vi "EV05故障解析.vi"() -> ()   [LabVIEW 2013]
panel:
  in  "选择故障类型":u32(ring) items=["电池故障", "硬件故障", "电池系统故障1", "电池系统故障2"]
  in  "输入故障码":string
  in  "故码障解析123":bool
  out "电池故障":string[][](array[string])
  # "故障码解析"
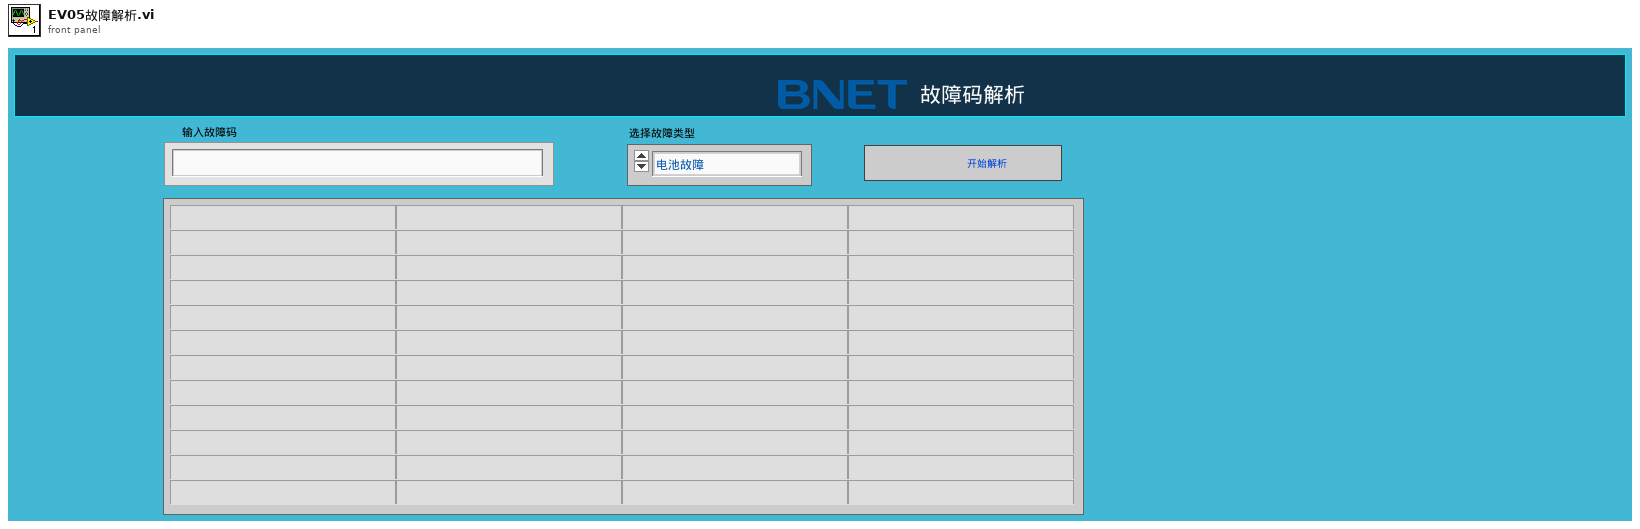
[diagram p1: front panel]
types:
  T1 = enum32{"Invalid", "Standard", "Closed", "Hidden", "Minimized", "Maximized"}
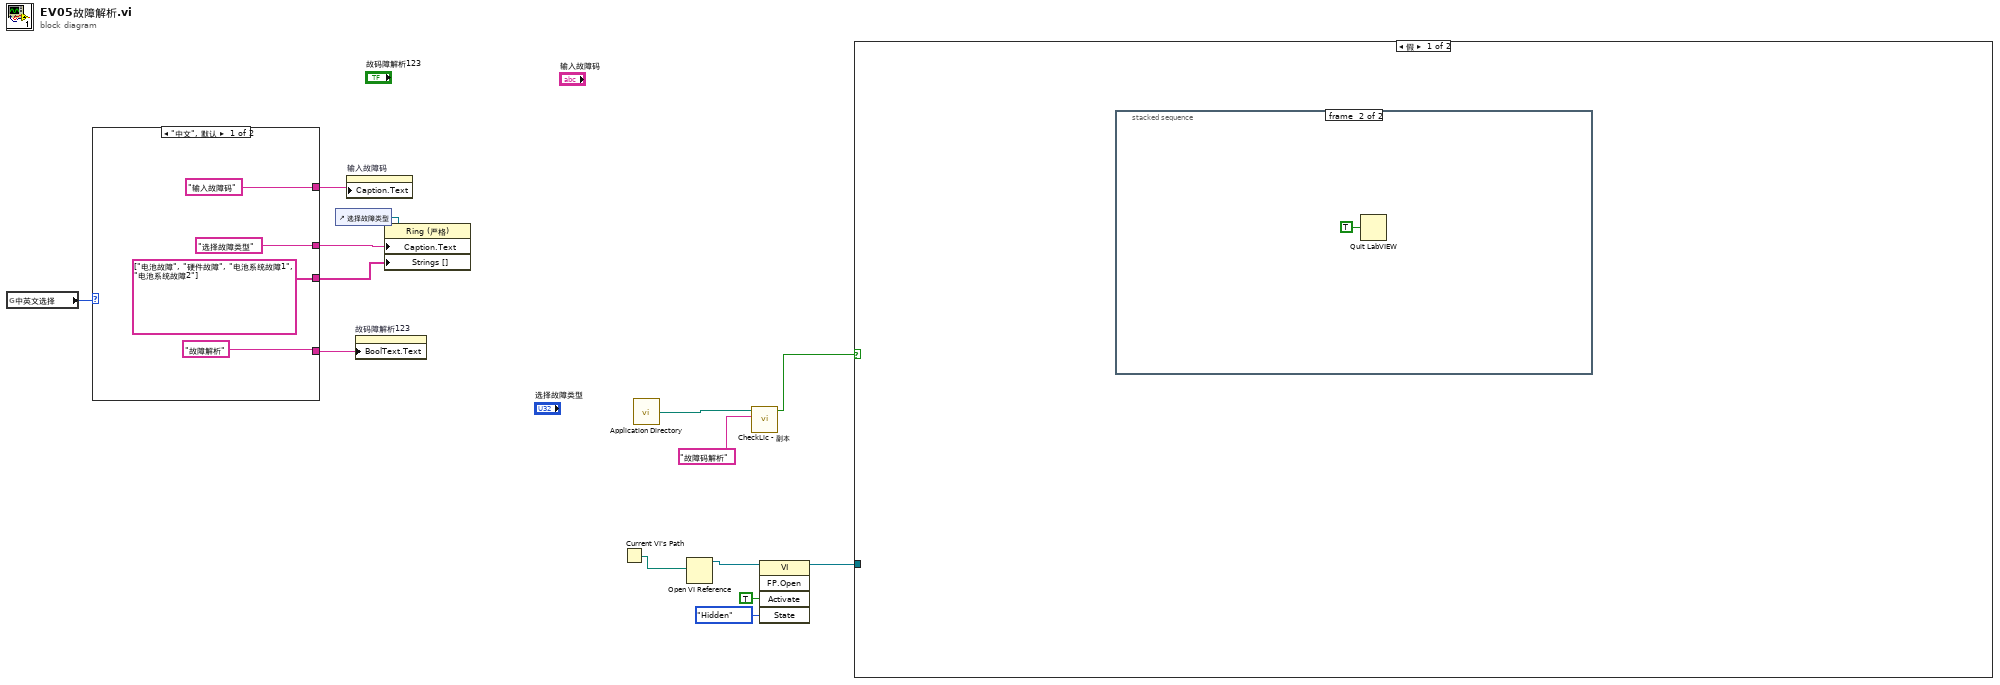
[diagram p0: block diagram]
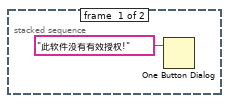
[diagram p2: hidden frame]
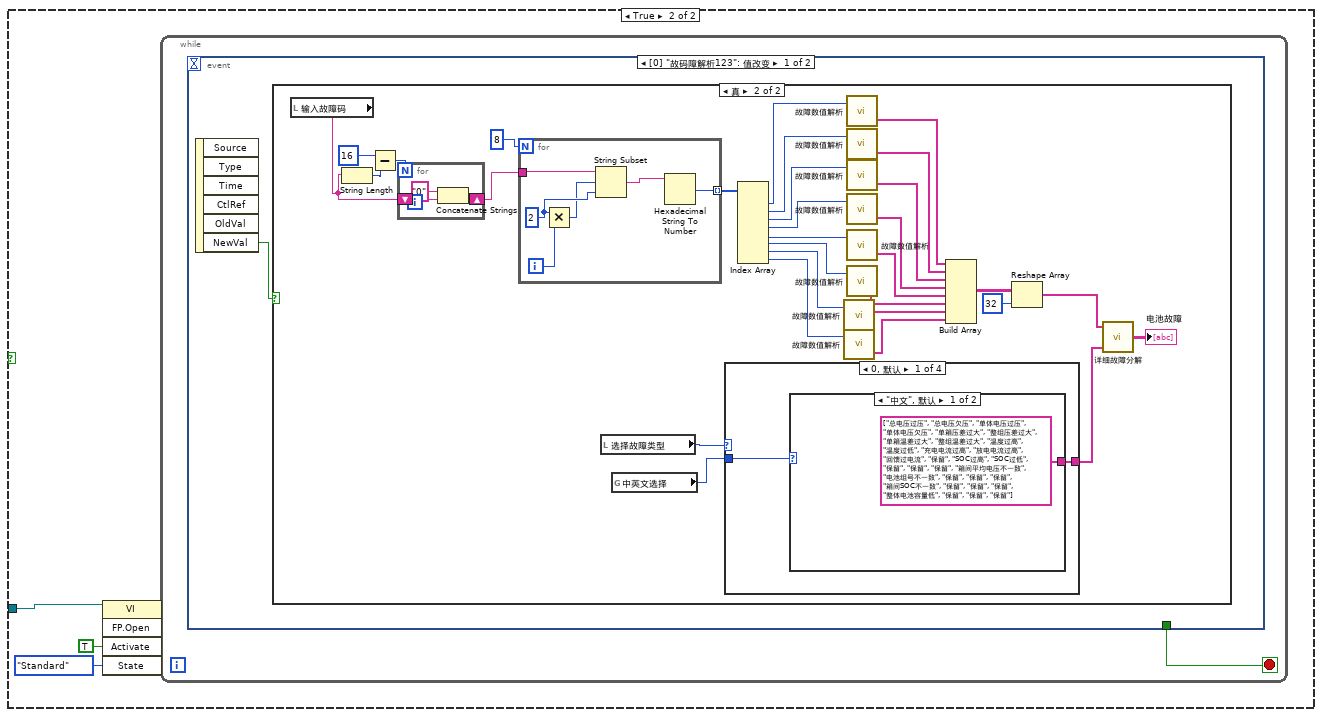
[diagram p3: hidden frame]
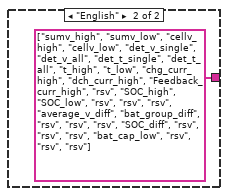
[diagram p5: hidden frame]
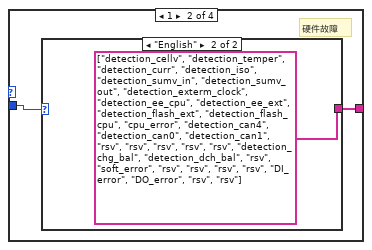
[diagram p6: hidden frame]
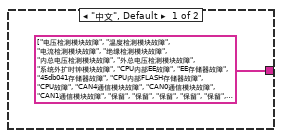
[diagram p7: hidden frame]
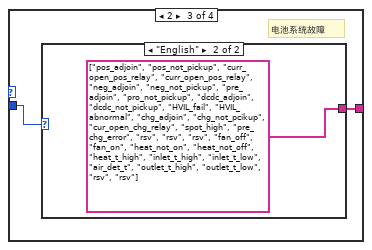
[diagram p8: hidden frame]
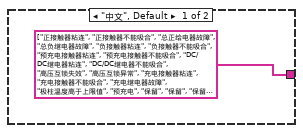
[diagram p9: hidden frame]
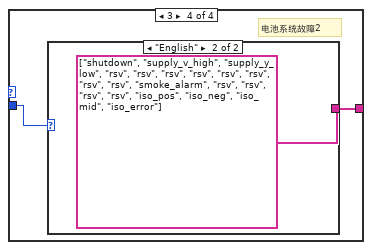
[diagram p10: hidden frame]
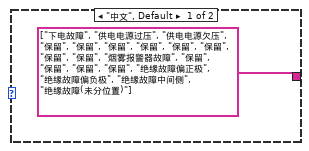
[diagram p11: hidden frame]
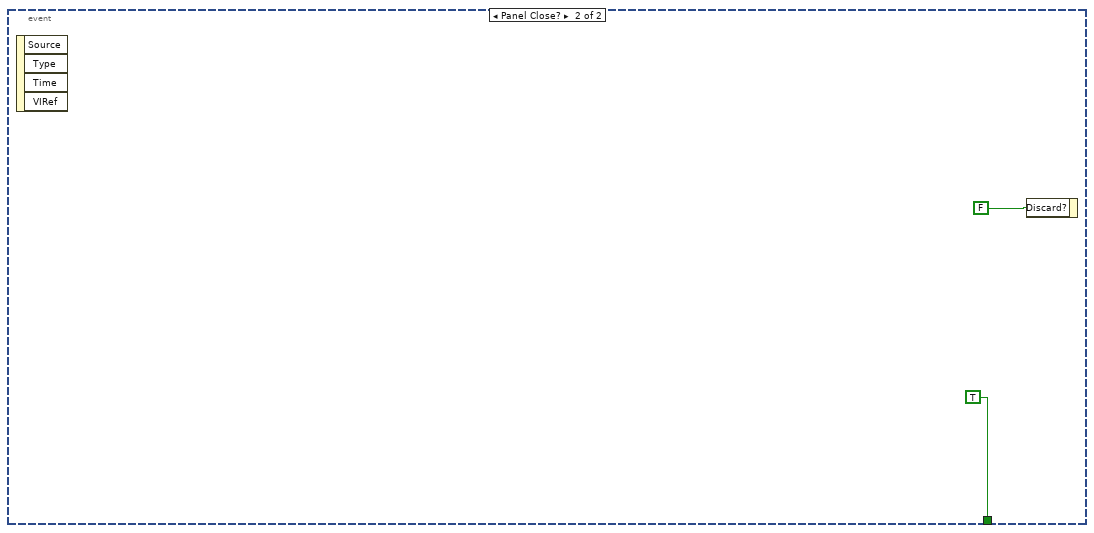
[diagram p12: hidden frame]
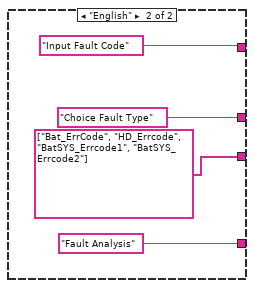
[diagram p13: hidden frame]
diagram:
  n1 = global read "中英文全局.vi" "中英文选择"() -> (w9:enum32{"中文", "English"})
  n2 = case shown="\"中文\", 默认" w9 {
    tunnel: ["输入故障码" "Input Fault Code"] -> w14
    tunnel: ["选择故障类型" "Choice Fault Type"] -> w12
    tunnel: [string[] ["电池故障", "硬件故障", "电池系统故障1", "电池系统故障2"] ("字符串[]") string[] ["Bat_ErrCode", "HD_Errcode", "BatSYS_Errcode1", "BatSYS_Errcode2"] ("字符串[]")] -> w11
    tunnel: ["故障解析" "Fault Analysis"] -> w10
    frame "中文", Default {
    }
    frame "English" {
    }
  }
  n3 = control-ref of="选择故障类型"() -> (w13:refnum<vi>)
  n4 = property on="输入故障码" class="Str"("Caption.Text"=w14) -> ()  [unwired: 2 in, 2 out]
  n5 = property on="故码障解析123" class="Bool (严格)"("BoolText.Text"=w10) -> ()  [unwired: 2 in, 2 out]
  n6 = property class="Ring (严格)"(reference=w13, "Caption.Text"=w12, "Strings []"=w11) -> ()  [unwired: 1 in, 2 out]
  n7 = Current VI's Path() -> (path=w6:path)
  n8 = call <vilib>:"Application Directory.vi"() -> ("Application Directory"=w7:path)
  n9 = Open VI Reference(vi path=w6) -> (vi reference=w5:refnum<vi>)  [unwired: 5 in, 1 out]
  n10 = call "CheckLic - 副本.vi"("路径"=w7, "对外文件夹名称"="故障码解析") -> ("鉴权通过"=w2:bool)  [unwired: 6 in]
  n11 = invoke class="VI" method="FP.Open"(reference=w5, "Activate"=TRUE ("激活？"), "State"=T1."Hidden" ("状态")) -> (reference out=w1:refnum<vi>)  [unwired: 2 in, 4 out]
  n12 = case shown="假" w2 {
    tunnel: w1 -> [_ w25]
    frame False {
      n13 = stacked-sequence {
        frame #0 {
          n14 = One Button Dialog(message="此软件没有有效授权!" ("消息")) -> ()  [unwired: 1 in, 1 out]
        }
        frame #1 {
          n15 = Quit LabVIEW(quit? (T)=TRUE ("退出？(T)")) -> ()
        }
      }
    }
    frame True {
      n16 = invoke class="VI" method="FP.Open"(reference=w25, "Activate"=TRUE ("激活？"), "State"=T1."Standard" ("状态")) -> ()  [unwired: 2 in, 5 out]
      n17 = while {
        stop <- w28 stop-if-true
        n18 = event shown="[0] \"故码障解析123\": 值改变" {
          selector: _ -> [_ _]
          dyn-events: _ -> [_ _]
          timeout: _ -> [_ _]
          tunnel: [_ TRUE] -> w28
          event "故码障解析123": Value Change {
            n19 = event-data() -> ("NewVal"=w29:bool)  [unwired: 1 in, 5 out]
            n20 = case shown="真" w29 {
              frame False {
              }
              frame True {
                n21 = local read "输入故障码"() -> (w32:string)
                n22 = String Length(string=w32) -> (length=w34:i32)
                n23 = Subtract(x=16, y=w34) -> (x-y=w36:i32)
                n24 = for {
                  N: w36 -> [_]
                  shift-right: [w60] -> w33
                  shift-left: w32 -> [w62]
                  n25 = Concatenate Strings("0" ("字符串"), w62) -> (w60:string)
                }
                n26 = for {
                  N: 8 -> [_]
                  tunnel: w33 -> [w68]
                  tunnel: [w67] -> w47 mode=indexing
                  i -> [w63]
                  w65 = 2 ("x")
                  n27 = Multiply(x=w65, y=w63) -> (x*y=w64:i32)
                  n28 = String Subset(string=w68, offset (0)=w64, length (rest)=w65) -> (substring=w66:string)
                  n29 = Hexadecimal String To Number(string=w66) -> (number=w67:u32)  [unwired: 2 in, 1 out]
                }
                n30 = local read "选择故障类型"() -> (w31:u32)
                n31 = global read "中英文全局.vi" "中英文选择"() -> (w30:enum32{"中文", "English"})
                n32 = case shown="0, 默认" w31 {
                  tunnel: [w70 w74 w78 w82] -> w59
                  tunnel: w30 -> [w69 w73 w77 w81]
                  frame 0, Default {
                    n33 = case shown="\"中文\", 默认" w69 {
                      tunnel: [string[] ["总电压过压", "总电压欠压", "单体电压过压", "单体电压欠压", "单箱压差过大", "整组压差过大", "单箱温差过大", "整组温差过大", "温度过高", "温度过低", "充电电流过高", "放电电流过高", "回馈过电流", "保留", "SOC过高", "SOC过低", "保留", "保留", "保留", "箱间平均电压不一致", "电池组号不一致", "保留", "保留", "保留", "箱间SOC不一致", "保留", "保留", "保留", "整体电池容量低", "保留", "保留", "保留"] ("名称") string[] ["sumv_high", "sumv_low", "cellv_high", "cellv_low", "det_v_single", "det_v_all", "det_t_single", "det_t_all", "t_high", "t_low", "chg_curr_high", "dch_curr_high", "Feedback_curr_high", "rsv", "SOC_high", "SOC_low", "rsv", "rsv", "rsv", "average_v_diff", "bat_group_diff", "rsv", "rsv", "rsv", "SOC_diff", "rsv", "rsv", "rsv", "bat_cap_low", "rsv", "rsv", "rsv"] ("名称")] -> w70
                      frame "中文", Default {
                      }
                      frame "English" {
                      }
                    }
                  }
                  frame 1 {
                    # "硬件故障"
                    n34 = case shown="\"English\"" w73 {
                      tunnel: [string[] ["电压检测模块故障", "温度检测模块故障", "电流检测模块故障", "绝缘检测模块故障", "内总电压检测模块故障", "外总电压检测模块故障", "系统外扩时钟模块故障", "CPU内部EE故障", "EE存储器故障", "45db041存储器故障", "CPU内部FLASH存储器故障", "CPU故障", "CAN4通信模块故障", "CAN0通信模块故障", "CAN1通信模块故障", "保留", "保留", "保留", "保留", "保留", "充电均衡模块故障", "放电均衡模块故障", "保留", "软件故障", "保留", "保留", "保留", "保留", "DI模块故障", "DO模块故障", "保留", "保留"] ("名称") string[] ["detection_cellv", "detection_temper", "detection_curr", "detection_iso", "detection_sumv_in", "detection_sumv_out", "detection_exterm_clock", "detection_ee_cpu", "detection_ee_ext", "detection_flash_ext", "detection_flash_cpu", "cpu_error", "detection_can4", "detection_can0", "detection_can1", "rsv", "rsv", "rsv", "rsv", "rsv", "detection_chg_bal", "detection_dch_bal", "rsv", "soft_error", "rsv", "rsv", "rsv", "rsv", "DI_error", "DO_error", "rsv", "rsv"] ("名称")] -> w74
                      frame "中文", Default {
                      }
                      frame "English" {
                      }
                    }
                  }
                  frame 2 {
                    # "电池系统故障"
                    n35 = case shown="\"English\"" w77 {
                      tunnel: [string[] ["正接触器粘连", "正接触器不能吸合", "总正给电器故障", "总负继电器故障", "负接触器粘连", "负接触器不能吸合", "预充电接触器粘连", "预充电接触器不能吸合", "DC/DC继电器粘连", "DC/DC继电器不能吸合", "高压互锁失效", "高压互锁异常", "充电接触器粘连", "充电接触器不能吸合", "充电继电器故障", "极柱温度高于上限值", "预充电", "保留", "保留", "保留", "风机堵路", "风机开路", "加热不能开启", "加热不能关闭", "加热器温度高于上限值", "进风口温度过高", "进风口温度过低", "进风口,出风口温差故障", "出风口温度过高", "出风口温度过低", "保留", "保留"] ("名称") string[] ["pos_adjoin", "pos_not_pickup", "curr_open_pos_relay", "curr_open_pos_relay", "neg_adjoin", "neg_not_pickup", "pre_adjoin", "pro_not_pickup", "dcdc_adjoin", "dcdc_not_pickup", "HVIL_fail", "HVIL_abnormal", "chg_adjoin", "chg_not_pcikup", "cur_open_chg_relay", "spot_high", "pre_chg_error", "rsv", "rsv", "rsv", "fan_off", "fan_on", "heat_not_on", "heat_not_off", "heat_t_high", "inlet_t_high", "inlet_t_low", "air_det_t", "outlet_t_high", "outlet_t_low", "rsv", "rsv"] ("名称")] -> w78
                      frame "中文", Default {
                      }
                      frame "English" {
                      }
                    }
                  }
                  frame 3 {
                    # "电池系统故障2"
                    n36 = case shown="\"English\"" w81 {
                      tunnel: [string[] ["下电故障", "供电电源过压", "供电电源欠压", "保留", "保留", "保留", "保留", "保留", "保留", "保留", "保留", "烟雾报警器故障", "保留", "保留", "保留", "保留", "绝缘故障偏正极", "绝缘故障偏负极", "绝缘故障中间侧", "绝缘故障(未分位置)"] ("名称") string[] ["shutdown", "supply_v_high", "supply_y_low", "rsv", "rsv", "rsv", "rsv", "rsv", "rsv", "rsv", "rsv", "smoke_alarm", "rsv", "rsv", "rsv", "rsv", "iso_pos", "iso_neg", "iso_mid", "iso_error"] ("名称")] -> w82
                      frame "中文", Default {
                      }
                      frame "English" {
                      }
                    }
                  }
                }
                n37 = Index Array(array=w47) -> (element #1=w46:u32, element #2=w45:u32, element #3=w44:u32, element #4=w43:u32, element #5=w42:u32, element #6=w41:u32, element #7=w40:u32, element #8=w39:u32)  [unwired: 8 in]
                n38 = call "故障数值解析.vi"("输入"=w40) -> ("结果"=w53:string[])  [unwired: 2 out]
                n39 = call "故障数值解析.vi"("输入"=w39) -> ("结果"=w51:string[])  [unwired: 2 out]
                n40 = call "故障数值解析.vi"("输入"=w46) -> ("结果"=w58:string[])  [unwired: 2 out]
                n41 = call "故障数值解析.vi"("输入"=w45) -> ("结果"=w57:string[])  [unwired: 2 out]
                n42 = call "故障数值解析.vi"("输入"=w44) -> ("结果"=w56:string[])  [unwired: 2 out]
                n43 = call "故障数值解析.vi"("输入"=w43) -> ("结果"=w52:string[])  [unwired: 2 out]
                n44 = call "故障数值解析.vi"("输入"=w42) -> ("结果"=w55:string[])  [unwired: 2 out]
                n45 = call "故障数值解析.vi"("输入"=w41) -> ("结果"=w54:string[])  [unwired: 2 out]
                n46 = Build Array(w58, w57, w56, w52, w55, w54, w53, w51) -> (w49:string[][])
                n47 = Reshape Array(w49, 32 ("维数大小")) -> (w48:string[])
                n48 = call "详细故障分解.vi"("名称"=w59, "故障输入口"=w48) -> ("输出数组"=→"电池故障":string[][])  [unwired: 3 out]
              }
            }
          }
          event Panel Close? {
            n49 = event-data() -> ()  [unwired: 1 in, 4 out]
            n50 = event-data("Discard?"=FALSE) -> ()  [unwired: 1 in, 1 out]
          }
        }
      }
    }
  }
